vi "ControlLED.vi"() -> ()   [LabVIEW 2020]
uses:
  rappg_lab3/Control 6.ctl
  <vilib>/DAQmx/write.llb/DAQmx Write (Digital 1D Bool 1Chan 1Samp).vi
  <vilib>/DAQmx/create/channels.llb/DAQmx Create Channel (DO-Digital Output).vi
  <vilib>/DAQmx/miscellaneous.llb/DAQmx Fill In Error Info.vi
panel:
  out "Enum":T1
  in  "LED Buttons 2":bool[](array[boolean])
  in  "stop":bool
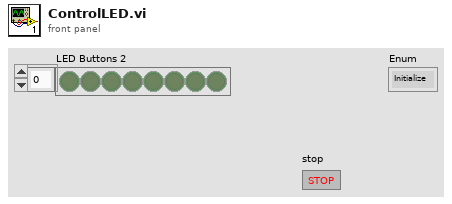
[diagram p1: front panel]
types:
  T1 = typedef "Control 6.ctl" = enum16{"Initialize", "Check for UI", "Stop"}
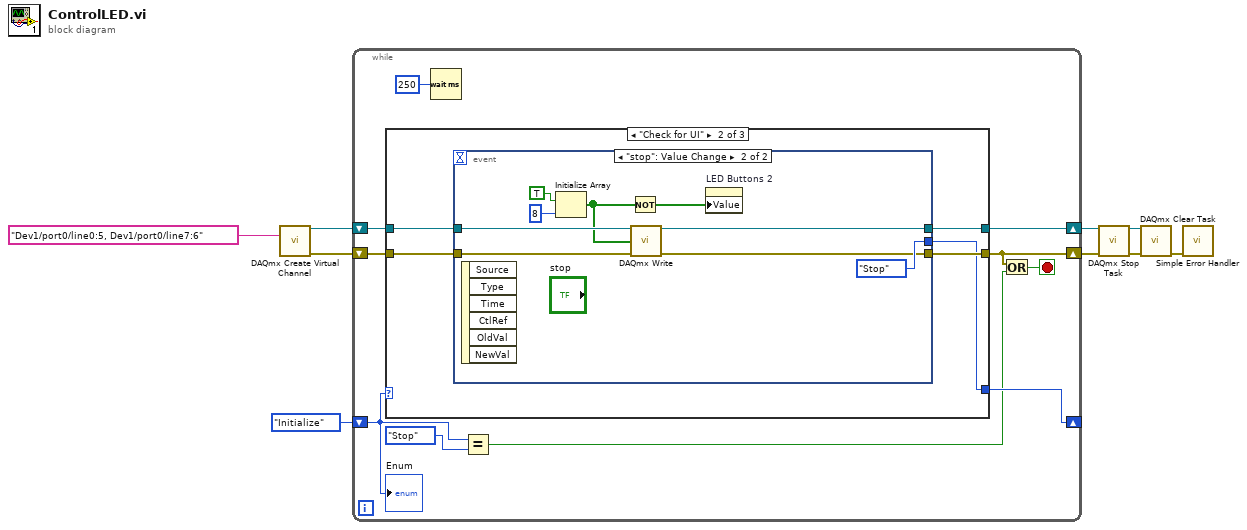
[diagram p0: block diagram]
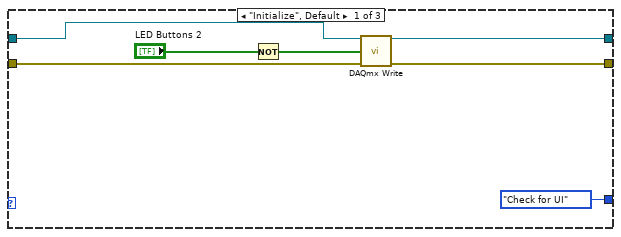
[diagram p2: hidden frame]
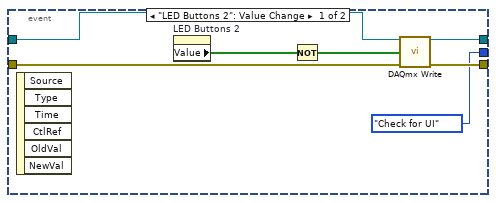
[diagram p3: hidden frame]
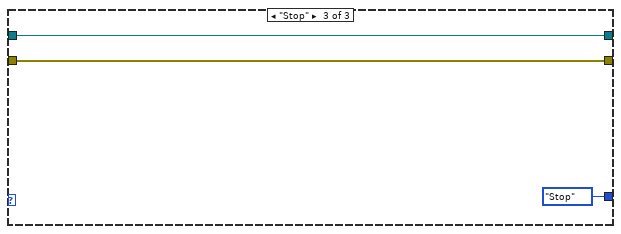
[diagram p4: hidden frame]
diagram:
  n1 = call-poly <vilib>:"DAQmx Create Virtual Channel.vi"("lines"=tag "Dev1/port0/line0:5, Dev1/port0/line7:6") -> ("task out"=w9:refnum<k21>, "error out"=w8:errorcluster)  [unwired: 13 in]
  n2 = while {
    shift-right: [w12] -> w6
    shift-left: w8 -> [w17]
    shift-right: [w16] -> w7
    shift-left: w9 -> [w18]
    shift-right: [w15] -> _
    shift-left: Control_6."Initialize" -> [w13]
    stop <- w10 stop-if-true
    n3 = case shown="\"Check for UI\"" w13 {
      tunnel: w18 -> [w26 w31 w49]
      tunnel: w17 -> [w25 w30 w48]
      tunnel: [w23 w29 w49] -> w16
      tunnel: [w24 w28 w48] -> w12
      tunnel: [Control_6."Check for UI" w27 Control_6."Stop"] -> w15
      frame "Initialize", Default {
        n4 = Not(x="LED Buttons 2") -> (.not. x?=w20:bool[])
        n5 = call-poly <vilib>:"DAQmx Write.vi"("task/channels in"=w26, "data"=w20, "error in"=w25) -> ("task out"=w23:refnum<k21>, "error out"=w24:errorcluster)  [unwired: 10 in, 1 out]
      }
      frame "Check for UI" {
        n6 = event shown="[1] \"stop\": Value Change" {
          selector: _ -> [_ _]
          dyn-events: _ -> [_ _]
          timeout: _ -> [_ _]
          tunnel: w31 -> [w38 w44]
          tunnel: w30 -> [w37 w43]
          tunnel: [w36 w42] -> w29
          tunnel: [w35 w41] -> w28
          tunnel: [Control_6."Check for UI" Control_6."Stop"] -> w27
          event "LED Buttons 2": Value Change {
            n7 = event-data() -> ()  [unwired: 1 in, 6 out]
            n8 = property on="LED Buttons 2" class="Arr (strict)"() -> ("Value"=w34:bool[])  [unwired: 2 in, 2 out]
            n9 = Not(x=w34) -> (.not. x?=w32:bool[])
            n10 = call-poly <vilib>:"DAQmx Write.vi"("task/channels in"=w38, "data"=w32, "error in"=w37) -> ("task out"=w36:refnum<k21>, "error out"=w35:errorcluster)  [unwired: 10 in, 1 out]
          }
          event "stop": Value Change {
            n11 = event-data() -> ()  [unwired: 1 in, 6 out]
            n12 = Initialize Array(TRUE, 8 ("dimension size")) -> (w40:bool[])
            n13 = Not(x=w40) -> (.not. x?=w39:bool[])
            n14 = call-poly <vilib>:"DAQmx Write.vi"("task/channels in"=w44, "data"=w40, "error in"=w43) -> ("task out"=w42:refnum<k21>, "error out"=w41:errorcluster)  [unwired: 10 in, 1 out]
            n15 = property on="LED Buttons 2" class="Arr (strict)"("Value"=w39) -> ()  [unwired: 2 in, 2 out]
          }
        }
      }
      frame "Stop" {
      }
    }
    n16 = Wait (ms)(milliseconds to wait=u32 250) -> ()  [unwired: 1 out]
    n17 = Equal?(x=w13, y=Control_6."Stop") -> (x = y?=w11:bool)
    n18 = Or(x=w12, y=w11) -> (x .or. y?=w10:bool)
    "Enum" <- w13
  }
  n19 = call <vilib>:"DAQmx Stop Task.vi"("task/channels in"=w7, "error in"=w6) -> ("task out"=w5:refnum<k21>, "error out"=w4:errorcluster)  [unwired: 12 in]
  n20 = call <vilib>:"DAQmx Clear Task.vi"("task in"=w5, "error in"=w4) -> ("error out"=w3:errorcluster)  [unwired: 13 in]
  n21 = call <vilib>:"Simple Error Handler.vi"("error in (no error)"=w3) -> ()  [unwired: 4 in, 5 out]
